vi "Write Visible.vi"(5 "Visible":bool, 9 "Decoration in":refnum<class "Decoration.lvclass">) -> (3 "Decoration out":refnum<class "Decoration.lvclass">)   [LabVIEW 2014, in "Raspberry Pi Compatible Compiler for LabVIEW.lvlib" / "Decoration.lvclass"]
uses:
  Decoration.lvclass
  Decoration.lvclass/Decoration.ctl
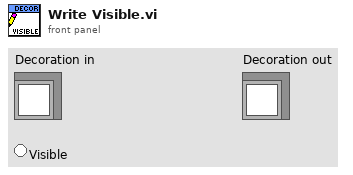
[diagram p1: front panel]
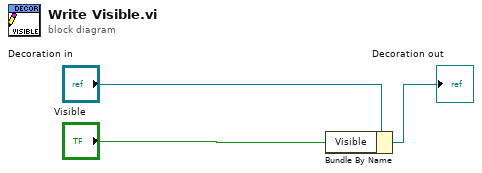
[diagram p0: block diagram]
diagram:
  n1 = Bundle By Name(cluster="Decoration in", "Visible"="Visible") -> (→"Decoration out":refnum<class "Decoration.lvclass">)
